vi "FFT_bkg removal.vi"(0 "Bfield":dbl[](array[numeric]), 2 "bkg removal method":enum16{"polynomial", "Cheby poly"}(ring), 3 "poly. order":i32=6, 5 "Data":dbl[](array[numeric]), 7 "B initial":dbl=31.0 format="%.2f", 9 "inverse":bool=TRUE, 11 "B final":dbl=31.0 format="%.2f", 12 "Bbkg initial":dbl=13.5 format="%.2f", 14 "Bbkg final":dbl=31.0 format="%.2f") -> (4 "extended data":dbl[](array[numeric]), 6 "XY Graph":cluster{"Bfield":dbl[], "Data":dbl[]}[](graph), 10 "extended B":dbl[](array[numeric]))   [LabVIEW 2024]
uses:
  <vilib>/Analysis/6fits.llb/Curve Fitting Criteria.ctl
  <vilib>/Analysis/NI_AALPro.lvlib
panel:
  in  "method":T1 items=["Least Square", "Least Absolute Residual", "Bisquare"]
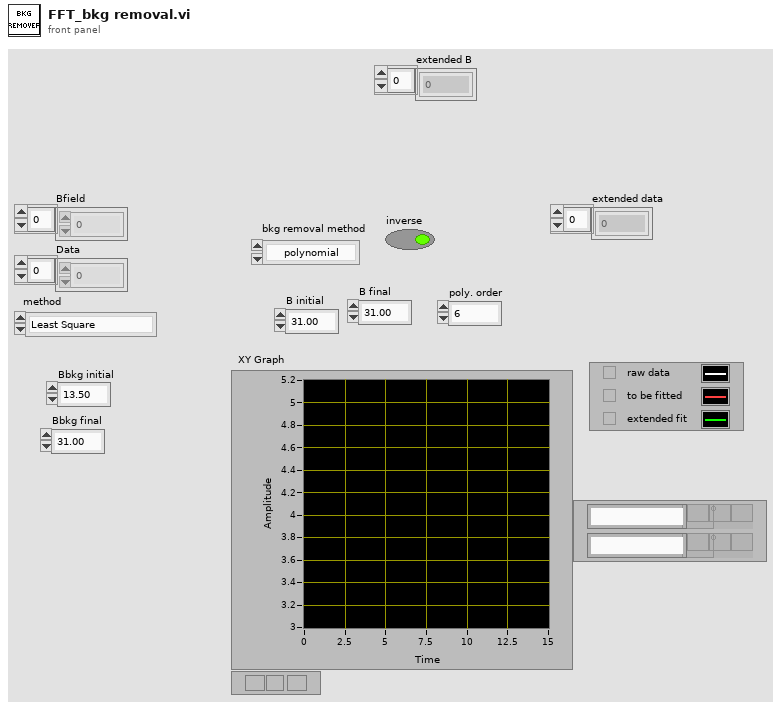
[diagram p1: front panel]
types:
  T1 = typedef "NI_AALPro.lvlib/Curve Fitting Criteria.ctl" = u16
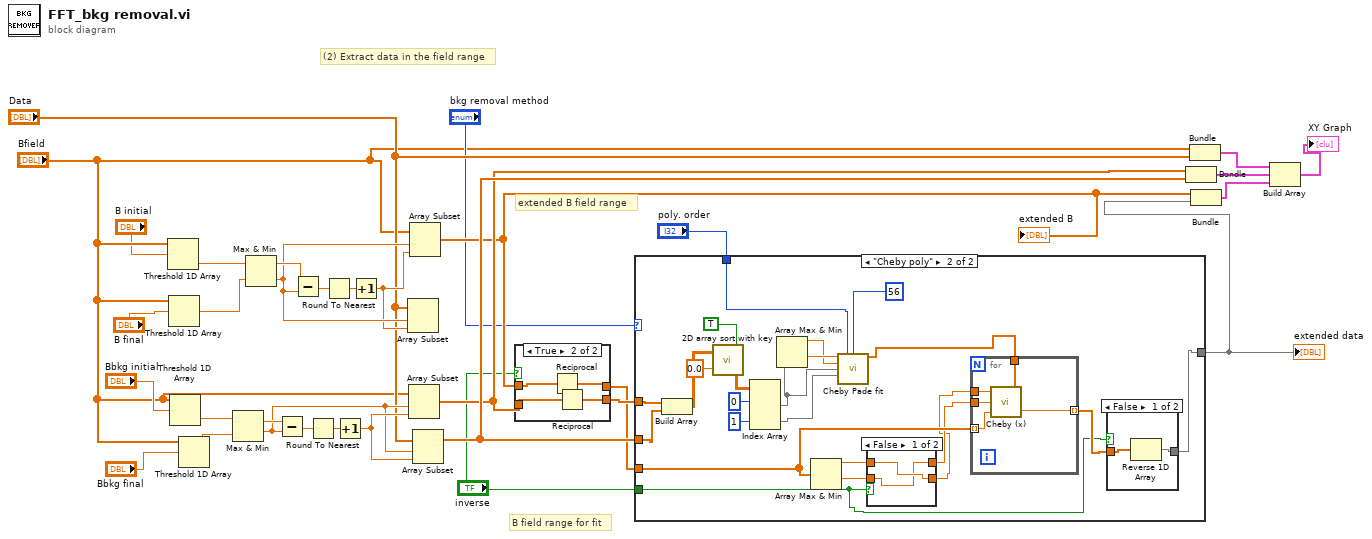
[diagram p0: block diagram]
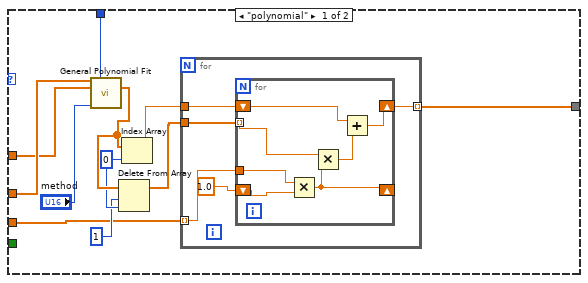
[diagram p3: hidden frame]
diagram:
  # "B field range for fit"
  # "extended B field range"
  # "(2) Extract data in the field range"
  n1 = Threshold 1D Array(2:"B initial", 3:"Bfield") -> (0:w1:dbl)  [unwired: 1 in]
  n2 = Threshold 1D Array(2:"B final", 3:"Bfield") -> (0:w10:dbl)  [unwired: 1 in]
  n3 = Threshold 1D Array(2:"Bbkg initial", 3:"Bfield") -> (0:w9:dbl)  [unwired: 1 in]
  n4 = Threshold 1D Array(2:"Bbkg final", 3:"Bfield") -> (0:w25:dbl)  [unwired: 1 in]
  n5 = Max & Min(x=w9, y=w25) -> (max(x,y)=w21:dbl, min(x,y)=w20:dbl)
  n6 = Max & Min(x=w1, y=w10) -> (max(x,y)=w32:dbl, min(x,y)=w30:dbl)
  n7 = Subtract(x=w21, y=w20) -> (x-y=w23:dbl)
  n8 = Subtract(x=w32, y=w30) -> (x-y=w31:dbl)
  n9 = Round To Nearest(number=w23) -> (nearest integer value=w24:dbl)
  n10 = Round To Nearest(number=w31) -> (nearest integer value=w33:dbl)
  n11 = Increment(x=w24) -> (x+1=w22:dbl)
  n12 = Increment(x=w33) -> (x+1=w28:dbl)
  n13 = Array Subset(array="Data", index=w30, length=w28) -> ()  [unwired: 1 out]
  n14 = Array Subset(array="Bfield", index=w20, length=w22) -> (w12:dbl[])
  n15 = Array Subset(array="Bfield", index=w30, length=w28) -> (w7:dbl[])
  "extended B" <- w7
  n16 = Array Subset(array="Data", index=w20, length=w22) -> (w18:dbl[])
  n17 = case shown="True" "inverse" {
    tunnel: [w35 w38] -> w11
    tunnel: w12 -> [w35 w39]
    tunnel: [w34 w36] -> w8
    tunnel: w7 -> [w34 w37]
    frame False {
    }
    frame True {
      n18 = Reciprocal(x=w37) -> (1/x=w36:dbl[])
      n19 = Reciprocal(x=w39) -> (1/x=w38:dbl[])
    }
  }
  n20 = case shown="\"Cheby poly\"" "bkg removal method" {
    tunnel: w18 -> [w50 w84]
    tunnel: w11 -> [w42 w85]
    tunnel: [w44 w64] -> w14
    tunnel: w8 -> [w41 w70]
    tunnel: "poly. order" -> [w40 w71]
    tunnel: "inverse" -> [_ w63]
    frame "polynomial" {
      w47 = 0 ("index")
      n21 = call <vilib>:"General Polynomial Fit.vi"("Y"=w50, "polynomial order"=w40, "X"=w42, "method"="method") -> ("Polynomial Coefficients"=w48:dbl[])  [unwired: 8 in, 3 out]
      n22 = Delete From Array(array=w48, length=1, index=w47) -> (array with subset deleted=w45:dbl[])  [unwired: 1 out]
      n23 = Index Array(array=w48, index=w47) -> (element=w43:dbl)
      n24 = for {
        tunnel: w45 -> [w54]
        tunnel: [w53] -> w44 mode=indexing
        tunnel: w43 -> [w52]
        tunnel: w41 -> [w51] mode=indexing
        n25 = for {
          tunnel: w54 -> [w60] mode=indexing
          shift-right: [w61] -> _
          shift-left: 1.0 -> [w62]
          shift-right: [w58] -> w53
          shift-left: w52 -> [w57]
          tunnel: w51 -> [w56]
          n26 = Multiply(x=w56, y=w62) -> (x*y=w61:dbl)
          n27 = Multiply(x=w60, y=w61) -> (x*y=w59:dbl)
          n28 = Add(x=w57, y=w59) -> (x+y=w58:dbl)
        }
      }
    }
    frame "Cheby poly" {
      n29 = Build Array(w85, w84) -> (w83:dbl[][])
      n30 = call "2D array sort with key.vi"("ascending"=TRUE, "key row"=0.0, "input"=w83) -> ("output"=w80:dbl[][])
      n31 = Index Array(array=w80, index (row) #1=0 ("index (row)"), index (row) #2=1 ("index (row)")) -> (element #1=w76:dbl[], element #2=w77:dbl[])  [unwired: 2 in]
      n32 = Array Max & Min(array=w76) -> (max value=w74:dbl, min value=w75:dbl)  [unwired: 2 out]
      n33 = Array Max & Min(array=w70) -> (max value=w69:dbl, min value=w67:dbl)  [unwired: 2 out]
      n34 = call "Cheby Pade fit.vi"("start"=w75, "order"=w71, "number of points"=u32 56, "end"=w74, "X-array"=w76, "Y-array"=w77) -> ("Tn coeffs"=w73:dbl[])  [unwired: 6 in, 3 out]
      n35 = case shown="False" w63 {
        tunnel: w69 -> [w90 w92]
        tunnel: [w89 w92] -> w68
        tunnel: w67 -> [w89 w91]
        tunnel: [w90 w91] -> w66
        frame False {
        }
        frame True {
        }
      }
      n36 = for {
        tunnel: w66 -> [w97]
        tunnel: w68 -> [w96]
        tunnel: w70 -> [w95] mode=indexing
        tunnel: w73 -> [w94]
        tunnel: [w93] -> w65 mode=indexing
        n37 = call "Cheby (x).vi"("Tn coeffs"=w94, "x"=w95, "end"=w96, "start"=w97) -> ("f(x)"=w93:dbl)
      }
      n38 = case shown="False" w63 {
        tunnel: w65 -> [w87 w88]
        tunnel: [w86 w88] -> w64
        frame False {
          n39 = Reverse 1D Array(array=w87) -> (reversed array=w86:dbl[])
        }
        frame True {
        }
      }
    }
  }
  "extended data" <- w14
  n40 = Bundle(w12, w18) -> (w16:cluster{dbl[], dbl[]})  [unwired: 1 in]
  n41 = Bundle("Bfield"="Bfield", "Data"="Data") -> (w17:cluster{"Bfield":dbl[], "Data":dbl[]})  [unwired: 1 in]
  n42 = Bundle(w7, w14) -> (w13:cluster{dbl[], dbl[]})  [unwired: 1 in]
  n43 = Build Array(w17, w16, w13) -> (→"XY Graph":cluster{"Bfield":dbl[], "Data":dbl[]}[])
